vi "cupFinderv5.vi"(11 "image\n in":T1(plugin-control)) -> (0 "WORK FOR GODS SAKE 2":T1(plugin-control), 1 "X-Out":dbl, 2 "CupPosition":T1(plugin-control), 3 "Refnum out":T1(plugin-control), 4 "Y-Out":dbl, 5 "ImgToCrop":T1(plugin-control))   [LabVIEW 2017]
uses:
  <vilib>/vision/NI_Vision_Development_Module.lvlib
panel:
  out "ROI Descriptor":T2 {"Contours"."Type" items=["No Selection", "Point", "Line", "Rectangle", "Oval", "Polygon", "Freehand Region", "Annulus", "Unused2", "Unused3", "Broken Line", "Freehand Line", "Rotated Rectangle"]}
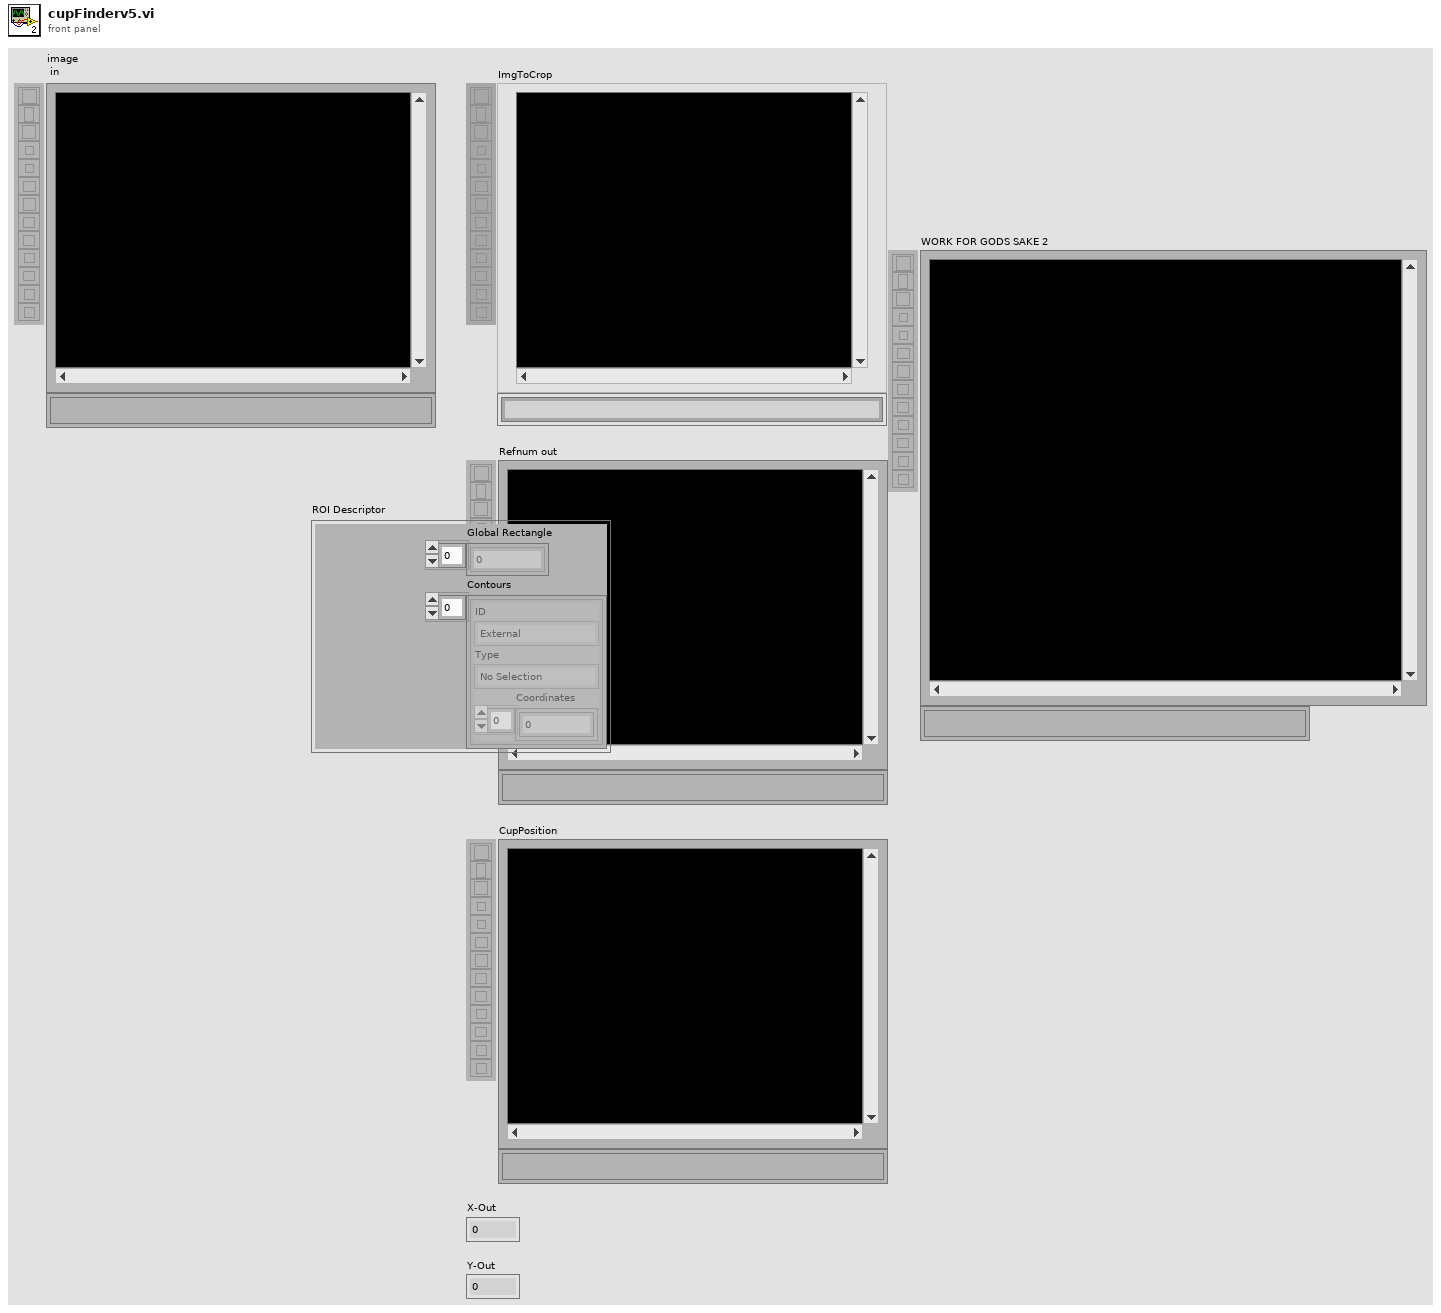
[diagram p1: front panel]
types:
  T1 = typedef "IMAQ Image.ctl" = refnum<image>
  T2 = cluster{"Global Rectangle":i32[], "Contours":cluster{"ID":enum32{"External", "Internal"}, "Type":u32, "Coordinates":i32[]}[]}
  T3 = typedef "Image Type" = u32
  T4 = cluster{"Position":cluster{"x":sgl, "y":sgl}, "Angle":sgl, "Scale":sgl, "Score":sgl, "Bounding Box":cluster{"x":sgl, "y":sgl}[]}[]
  T5 = typedef "IMAQ Rectangle" = cluster{"Left":i32, "Top":i32, "Right":i32, "Bottom":i32, "Rotation":dbl}
  T6 = typedef "ROI Descriptor" = cluster{"Global Rectangle":i32[], "Contours":cluster{"ID":enum32{"External", "Internal"}, "Type":u32, "Coordinates":i32[]}[]}
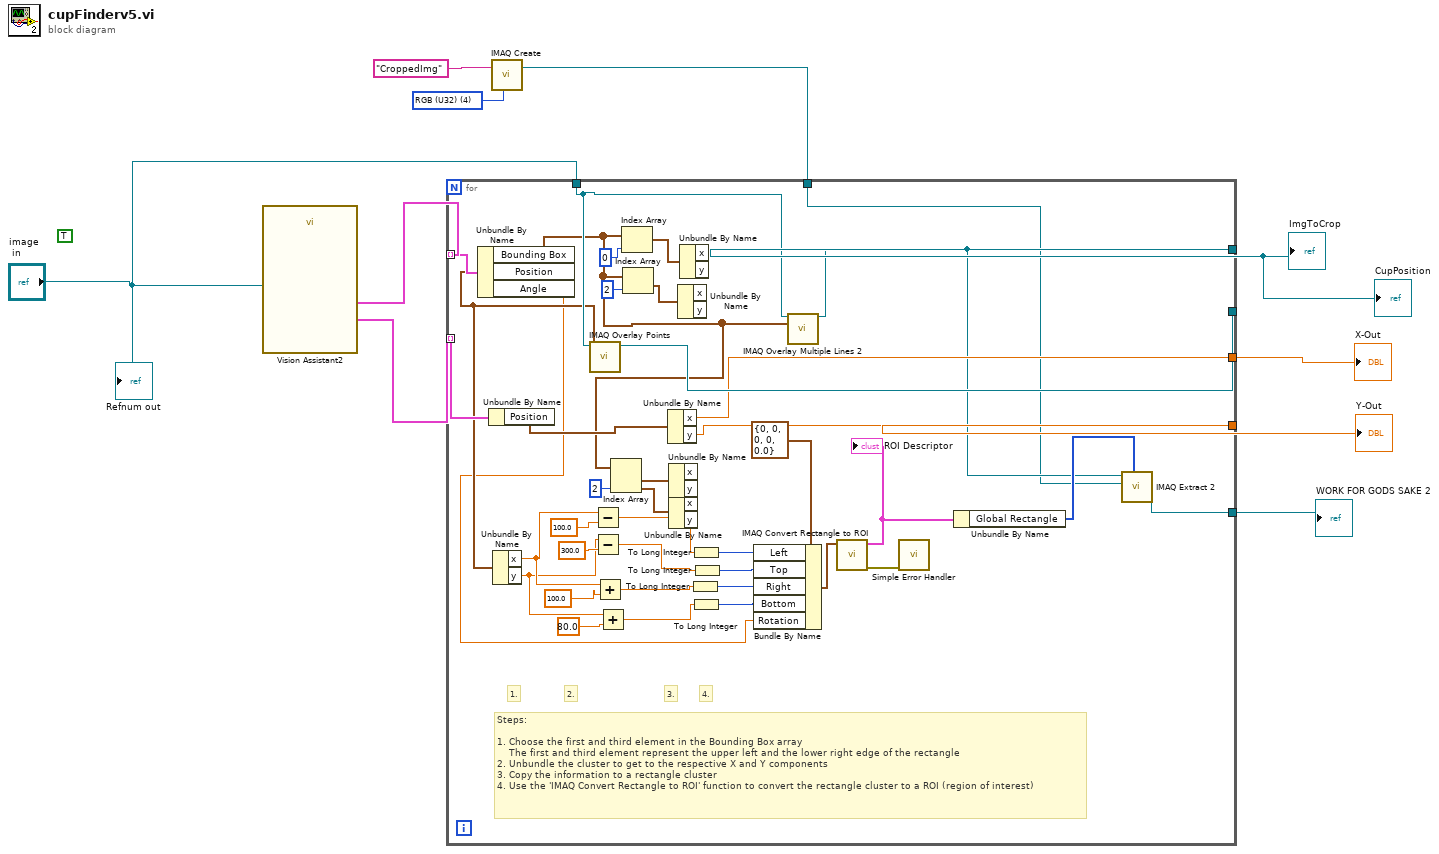
[diagram p0: block diagram]
diagram:
  w9 = T3 4 items=["Grayscale (U8)", "Grayscale (I16)", "Grayscale (SGL)", "Complex (CSG)", "RGB (U32)", "HSL (U32)", "RGB (U64)", "Grayscale (U16)"] ("Image Type")
  (unwired) TRUE
  n1 = call "Vision Assistant2"("Image In"="image\n in") -> ("Calibrated Matches (Pattern Matching 5)"=w2:T4, "Matches (Pattern Matching 5)"=w3:T4)  [unwired: 23 in, 2 out]
  n2 = call "IMAQ Create"("Image Name"="CroppedImg", "Image Type"=w9) -> ("New Image"=w10:T1)  [unwired: 3 in, 1 out]
  n3 = for {
    tunnel: [w25] -> w1
    tunnel: [w49] -> _
    tunnel: [w47] -> w6
    tunnel: [w46] -> w7
    tunnel: "image\n in" -> [w39]
    tunnel: w3 -> [w44] mode=indexing
    tunnel: w2 -> [w45] mode=indexing
    tunnel: w10 -> [w24]
    tunnel: [w23] -> w5
    # "1."
    # "2."
    # "3."
    # "4."
    # "Steps:\n\n1. Choose the first and third element in the Bounding Box array\n    The first and third element represent the upper left and the lower right edge of the rectangle\n2. Unbundle the cluster to get to the respective X and Y components\n3. Copy the information to a rectangle cluster\n4. Use the 'IMAQ Convert Rectangle to ROI' function to convert the rectangle cluster to a ROI (region of interest)"
    n4 = Unbundle By Name(w44) -> ("Bounding Box"=w26:cluster{"x":sgl, "y":sgl}[], "Position"=w22:cluster{"x":sgl, "y":sgl}, "Angle"=w11:sgl)
    n5 = Unbundle By Name(w45) -> ("Position"=w48:cluster{"x":sgl, "y":sgl})
    n6 = Unbundle By Name(w22) -> ("x"=w17:sgl, "y"=w14:sgl)
    n7 = call "IMAQ Overlay Points"("Point"=w22, "Image"=w39) -> ("Image Out"=w49:T1)  [unwired: 8 in, 1 out]
    n8 = Subtract(x=w17, y=sgl 100.0) -> (x-y=w20:sgl)
    n9 = Subtract(x=w14, y=sgl 300.0) -> (x-y=w18:sgl)
    n10 = Add(x=w17, y=sgl 100.0) -> (x+y=w15:sgl)
    n11 = Add(x=w14, y=sgl 80.0) -> (x+y=w12:sgl)
    n12 = Index Array(array=w26, index #2=2 ("index")) -> (element #1=w37:cluster{"x":sgl, "y":sgl}, element #2=w36:cluster{"x":sgl, "y":sgl})  [unwired: 1 in]
    n13 = Index Array(array=w26, index=0) -> (element=w42:cluster{"x":sgl, "y":sgl})
    n14 = Index Array(array=w26, index=2) -> (element=w40:cluster{"x":sgl, "y":sgl})
    n15 = Unbundle By Name(w48) -> ("x"=w47:sgl, "y"=w46:sgl)
    n16 = Unbundle By Name(w37) -> ()  [unwired: 2 out]
    n17 = Unbundle By Name(w36) -> ()  [unwired: 2 out]
    n18 = Unbundle By Name(w40) -> ()  [unwired: 2 out]
    n19 = Unbundle By Name(w42) -> ()  [unwired: 2 out]
    n20 = To Long Integer(number=w15) -> (32bit integer=w31:i32)
    n21 = To Long Integer(number=w20) -> (32bit integer=w33:i32)
    n22 = To Long Integer(number=w12) -> (32bit integer=w30:i32)
    n23 = To Long Integer(number=w18) -> (32bit integer=w32:i32)
    n24 = Bundle By Name(cluster=T5 {"Left"=0, "Top"=0, "Right"=0, "Bottom"=0, "Rotation"=0.0} ("Rectangle"), "Left"=w33, "Top"=w32, "Right"=w31, "Bottom"=w30, "Rotation"=w11) -> (w35:T5)
    n25 = call "IMAQ Overlay Multiple Lines 2"("Image"=w39, "Line End Points"=w26) -> ("Image Out"=w25:T1)  [unwired: 12 in, 1 out]
    n26 = call "IMAQ Convert Rectangle to ROI"("Rectangle"=w35) -> ("error out"=w29:errorcluster, "ROI Descriptor"=w28:T6)  [unwired: 8 in]
    "ROI Descriptor" <- w28
    n27 = call <vilib>:"Simple Error Handler.vi"("error in (no error)"=w29) -> ()  [unwired: 4 in, 5 out]
    n28 = Unbundle By Name(w28) -> ("Global Rectangle"=w27:i32[])
    n29 = call "IMAQ Extract 2"("Optional Rectangle"=w27, "Image Dst"=w24, "Image Src"=w25) -> ("Image Dst Out"=w23:T1)  [unwired: 7 in, 1 out]
  }
  "ImgToCrop" <- w1
  "CupPosition" <- w1
  "X-Out" <- w6
  "Y-Out" <- w7
  "WORK FOR GODS SAKE 2" <- w5
  "Refnum out" <- "image\n in"
